vi "RT Sims New.vi"() -> ()   [LabVIEW 2014]
uses:
  RT Streams Config.vi
  <resource>/objmgr/ni.dex.rc
panel:
  out "error out":errorcluster
  in  "Send Data":bool
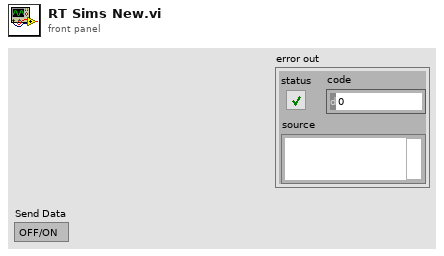
[diagram p1: front panel]
types:
  T1 = enum16{"Initialize", "Wait for Other", "Send Data"}
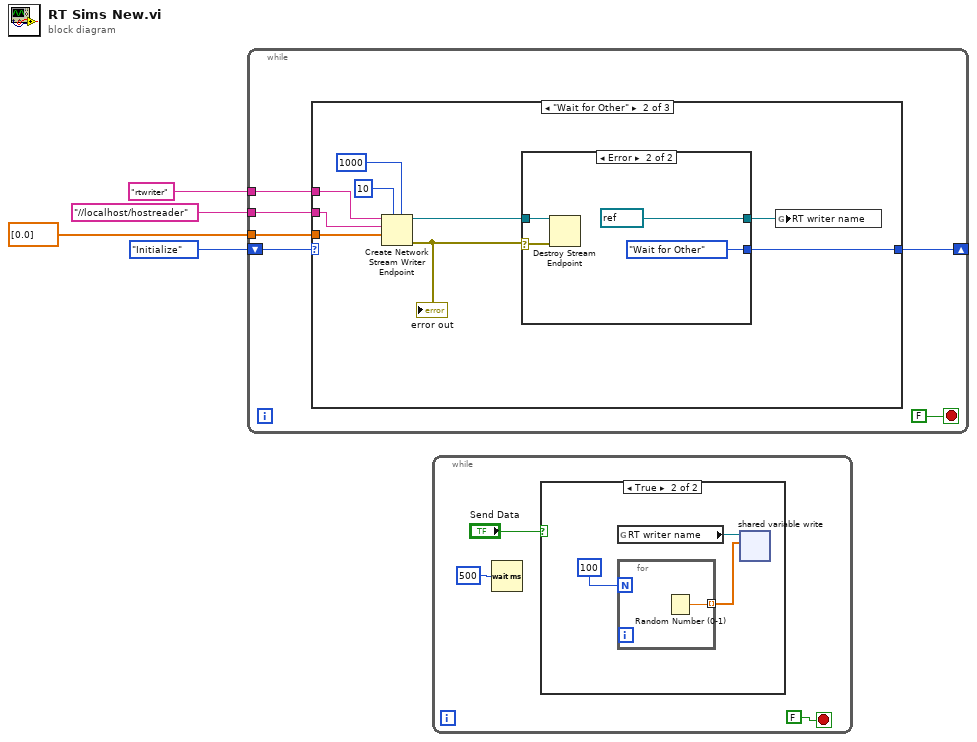
[diagram p0: block diagram]
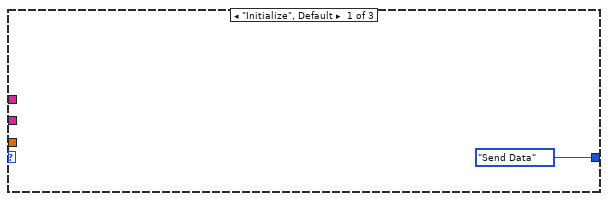
[diagram p3: hidden frame]
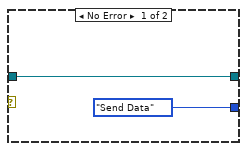
[diagram p4: hidden frame]
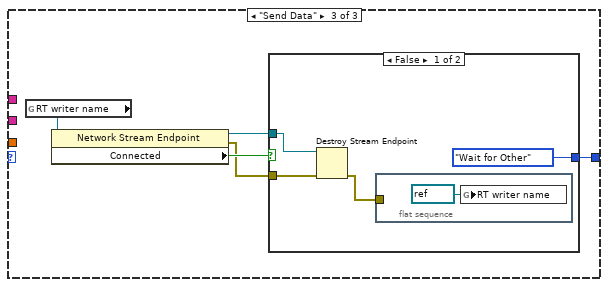
[diagram p5: hidden frame]
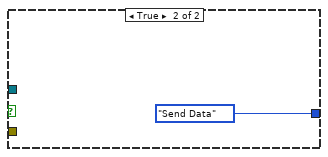
[diagram p6: hidden frame]
diagram:
  n1 = while {
    shift-right: [w8] -> _
    shift-left: T1."Initialize" -> [w10]
    tunnel: "rtwriter" ("writer name") -> [w7]
    tunnel: "//localhost/hostreader" ("reader url") -> [w6]
    tunnel: dbl[] [0.0] -> [w5]
    stop <- FALSE stop-if-true
    n2 = case shown="\"Wait for Other\"" w10 {
      tunnel: [T1."Send Data" w13 w29] -> w8
      tunnel: w7 -> [_ w20 _]
      tunnel: w6 -> [_ w19 _]
      tunnel: w5 -> [_ w12 _]
      frame "Initialize", Default {
      }
      frame "Wait for Other" {
        n3 = Create Network Stream Writer Endpoint(5:1000 ("timeout in ms (-1)"), 7:10 ("writer buffer size"), 9:w12, 10:w19, 11:w20) -> (0:w16:errorcluster, 3:w15:refnum<k21>)  [unwired: 2 in]
        "error out" <- w16
        n4 = case shown="Error" w16 {
          selector: w16 -> [_ w25]
          tunnel: w15 -> [w22 w26]
          tunnel: [w22 refnum<k21> refnum ("RT writer name")] -> w14
          tunnel: [T1."Send Data" T1."Wait for Other"] -> w13
          frame No Error {
          }
          frame Error {
            n5 = Destroy Stream Endpoint(8:w25, 11:w26) -> ()  [unwired: 1 out]
          }
        }
        n6 = global write "RT Streams Config.vi" "RT writer name"(w14) -> ()
      }
      frame "Send Data" {
        n7 = global read "RT Streams Config.vi" "RT writer name"() -> (w31:refnum<k21>)
        n8 = property class="Network Stream Endpoint"(reference=w31) -> (reference out=w28:refnum<k21>, error out=w27:errorcluster, "Connected"=w30:bool)  [unwired: 1 in]
        n9 = case shown="False" w30 {
          tunnel: [T1."Wait for Other" T1."Send Data"] -> w29
          tunnel: w28 -> [w34 _]
          tunnel: w27 -> [w33 _]
          frame False {
            n10 = Destroy Stream Endpoint(8:w33, 11:w34) -> (0:w32:errorcluster)
            n11 = flat-sequence {
              tunnel: w32 -> [_]
              frame #0 {
                n12 = global write "RT Streams Config.vi" "RT writer name"(refnum<k21> refnum ("RT writer name")) -> ()
              }
            }
          }
          frame True {
          }
        }
      }
    }
  }
  n13 = while {
    stop <- FALSE stop-if-true
    n14 = Wait (ms)(milliseconds to wait=u32 500) -> ()  [unwired: 1 out]
    n15 = case shown="True" "Send Data" {
      frame False {
      }
      frame True {
        n16 = global read "RT Streams Config.vi" "RT writer name"() -> (w43:refnum<k21>)
        n17 = for {
          N: 100 -> [_]
          tunnel: [w44] -> w42 mode=indexing
          n18 = Random Number (0-1)() -> (number: 0 to 1=w44:dbl)
        }
        n19 = shared-variable-write(w43, w42) -> ()  [unwired: 2 in, 3 out]
      }
    }
  }
